vi "9.6.vi"() -> ()   [LabVIEW 2019]
panel:
  out "prime?":bool
  in  "integer":dbl
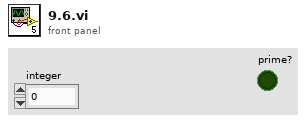
[diagram p1: front panel]
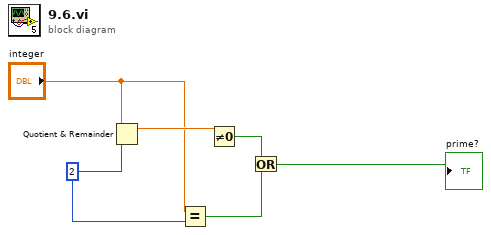
[diagram p0: block diagram]
diagram:
  w4 = 2
  n1 = Quotient & Remainder(x="integer", y=w4) -> (x-y*floor(x/y)=w6:dbl)  [unwired: 1 out]
  n2 = Equal?(x="integer", y=w4) -> (x = y?=w3:bool)
  n3 = Not Equal To 0?(x=w6) -> (x != 0?=w5:bool)
  n4 = Or(x=w5, y=w3) -> (x .or. y?=→"prime?":bool)
